vi "Write CIF Channel.vi"(8 "error in (no error)":errorcluster, 10 "CIF Channel":refnum<k21>, 11 "CIFTag in":refnum<class "CIF_NIChn.lvclass">) -> (0 "error out":errorcluster, 3 "CIFTag out":refnum<class "CIF_NIChn.lvclass">)   [LabVIEW 2021, in "CIF_NIChn.lvclass"]
uses:
  CIF_NIChn.lvclass
  CIF_NIChn.lvclass/CIF_NIChn.ctl
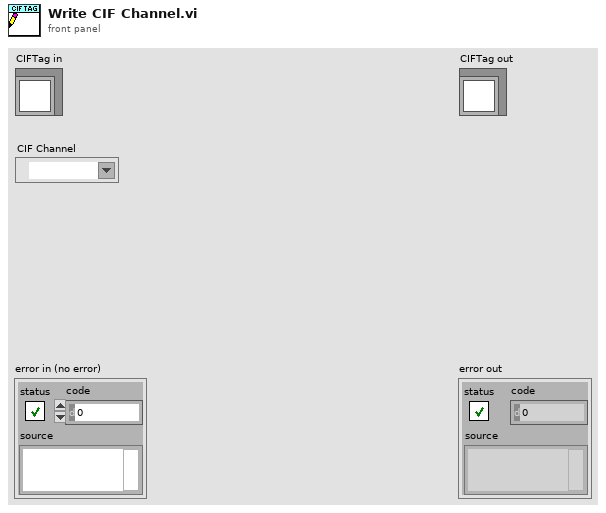
[diagram p1: front panel]
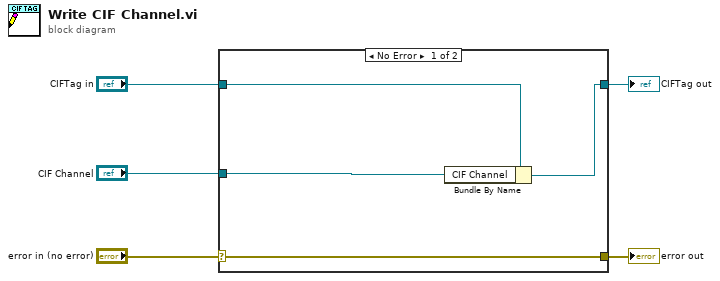
[diagram p0: block diagram]
diagram:
  n1 = case shown="No Error" "error in (no error)" {
    selector: "error in (no error)" -> [w9 w10]
    tunnel: [w9 w10] -> w4
    tunnel: [w7 w11] -> w2
    tunnel: "CIFTag in" -> [w8 w11]
    tunnel: "CIF Channel" -> [w6 _]
    frame No Error {
      n2 = Bundle By Name(cluster=w8, "CIF Channel"=w6) -> (w7:refnum<class "CIF_NIChn.lvclass">)
    }
    frame Error {
    }
  }
  "error out" <- w4
  "CIFTag out" <- w2
